vi "MAIN -- CREATE DOCS.vi"(7 "Project Root":path, 8 "error in (no error)":errorcluster, 9 "Demo Version":bool, 10 "Library Info Path":path, 11 "Target Folder":path) -> (0 "error out":errorcluster)   [LabVIEW 2011]
uses:
  <userlib>/_OpenG.lib/file/file.llb/Append Path to Root if Relative - Scalar__ogtk.vi
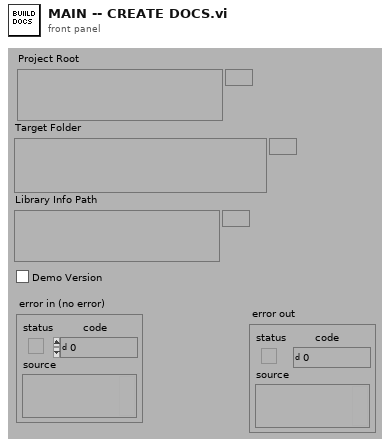
[diagram p1: front panel]
types:
  T1 = typedef "Library Information Cluster.ctl" = cluster{"Name":string, "Palette Submenu Image":path, "Palette Icon Image":path, "Description":string, "Documentation":string, "Installed Examples Folder":path, "Source Examples Folder":path, "Library VI":path[], "Installed Documentation Folder":path, "Product URL":string, "Info Email":string, "Copyright Notice":string, "Copyright Year":string}
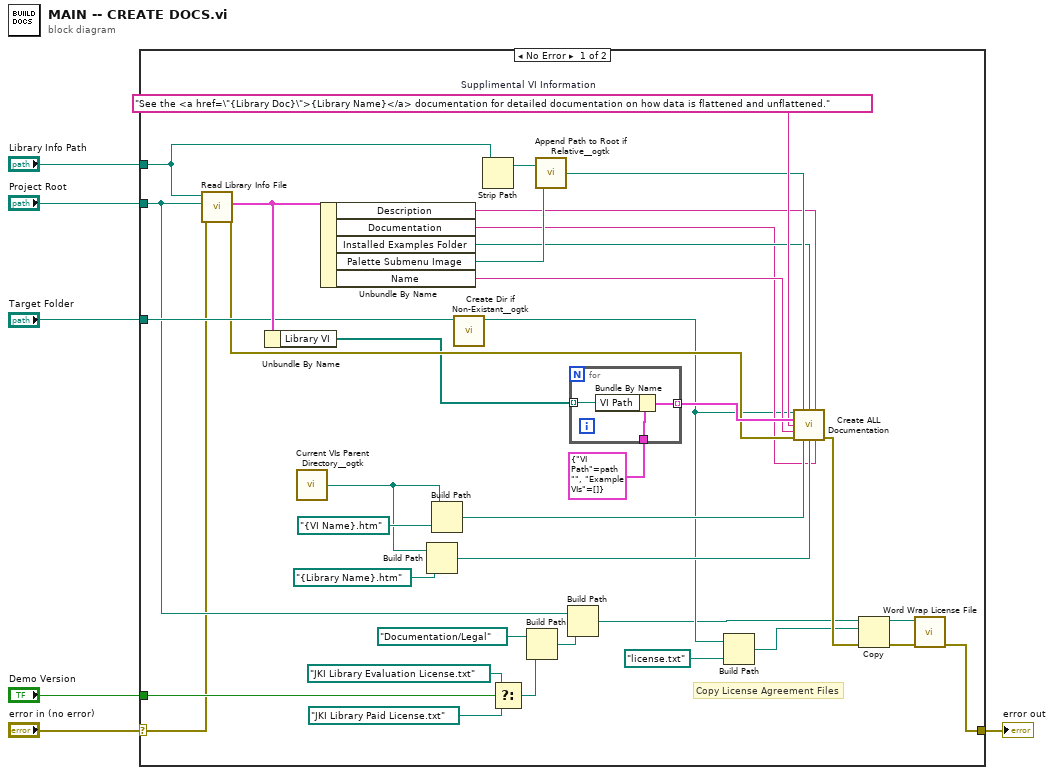
[diagram p0: block diagram]
diagram:
  n1 = case shown="No Error" "error in (no error)" {
    selector: "error in (no error)" -> [w7 w46]
    tunnel: "Library Info Path" -> [w38 _]
    tunnel: "Target Folder" -> [w28 _]
    tunnel: "Demo Version" -> [w15 _]
    tunnel: "Project Root" -> [w12 _]
    tunnel: [w9 w46] -> w2
    frame No Error {
      w40 = "See the <a href=\"{Library Doc}\">{Library Name}</a> documentation for detailed documentation on how data is flattened and unflattened."  # Supplimental VI Information
      # "Copy License Agreement Files"
      n2 = call "Read Library Info File.vi"("error in (no error)"=w7, "Project Root"=w12, "Library Info Path"=w38) -> ("error out"=w27:errorcluster, "Library Info"=w39:T1)  [unwired: 6 in, 1 out]
      n3 = Unbundle By Name(w39) -> ("Library VI"=w25:path[])
      n4 = call <userlib>:"Current VIs Parent Directory__ogtk.vi"() -> ("Parent Directory (+ Relative)"=w24:path)  [unwired: 5 in]
      n5 = Unbundle By Name(w39) -> ("Description"=w23:string, "Documentation"=w22:string, "Installed Examples Folder"=w29:path, "Palette Submenu Image"=w36:path, "Name"=w34:string)
      n6 = Build Path(base path=w24, name or relative path=path "{Library Name}.htm") -> (appended path=w32:path)
      n7 = Build Path(base path=w24, name or relative path=path "{VI Name}.htm") -> (appended path=w30:path)
      n8 = call <userlib>:"Create Dir if Non-Existant__ogtk.vi"("Directory Path"=w28) -> ("dup Directory Path"=w19:path)  [unwired: 8 in, 2 out]
      n9 = Strip Path(path=w38) -> (stripped path=w37:path)  [unwired: 1 out]
      n10 = Select(t=path "JKI Library Evaluation License.txt", s=w15, f=path "JKI Library Paid License.txt") -> (s? t:f=w14:path)
      n11 = Build Path(base path=path "Documentation/Legal", name or relative path=w14) -> (appended path=w13:path)
      n12 = call-poly <userlib>:"Append Path to Root if Relative__ogtk.vi"("Absolute or Relative Path"=w36, "Root Path"=w37) -> ("Absolute or Appended Path"=w35:path)
      n13 = Build Path(base path=w12, name or relative path=w13) -> (appended path=w11:path)
      n14 = for {
        tunnel: w25 -> [w44] mode=indexing
        tunnel: cluster{"VI Path":path, "Example VIs":string[]} {"VI Path"=path "", "Example VIs"=[]} ("VI Info") -> [w45]
        tunnel: [w43] -> w41 mode=indexing
        n15 = Bundle By Name(cluster=w45, "VI Path"=w44) -> (w43:cluster{"VI Path":path, "Example VIs":string[]})
      }
      n16 = Build Path(base path=w19, name or relative path=path "license.txt") -> (appended path=w18:path)
      n17 = call "Create ALL Documentation.vi"("Target Folder"=w19, "Library Palette Icon"=w35, "Library Examples Folder"=w29, "Library Description"=w23, "VI Paths"=w41, "Supplimental VI Information"=w40, "Library Name"=w34, "error in (no error)"=w27, "Template VI HTML Doc"=w30, "Template Library HTML Doc"=w32, "Library Documentation"=w22) -> ("error out"=w26:errorcluster)  [unwired: 4 in]
      n18 = Copy(8:w26, 10:w18, 11:w11) -> (0:w8:errorcluster, 3:w10:path)  [unwired: 2 in, 1 out]
      n19 = call "Word Wrap License File.vi"("error in"=w8, "txt file path"=w10) -> ("error out"=w9:errorcluster)  [unwired: 9 in]
    }
    frame Error {
    }
  }
  "error out" <- w2
